vi "Get Device Name.vi"(8 "error in (no error)":errorcluster, 11 "DeviceIndex":u32) -> (0 "error out":errorcluster, 3 "Device Name":string)   [LabVIEW 2014]
doc: "Gets the name of the device specified by <index>"
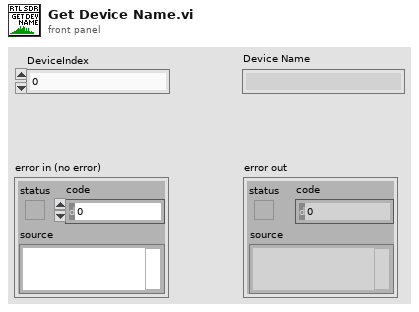
[diagram p1: front panel]
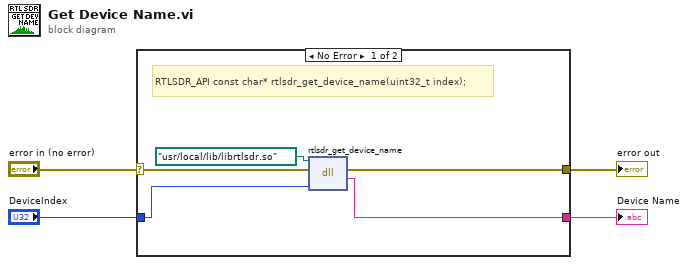
[diagram p0: block diagram]
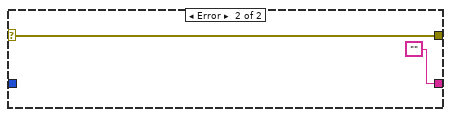
[diagram p2: hidden frame]
diagram:
  n1 = case shown="No Error" "error in (no error)" {
    selector: "error in (no error)" -> [w7 w10]
    tunnel: [w9 ""] -> w4
    tunnel: "DeviceIndex" -> [w8 _]
    tunnel: [w5 w10] -> w1
    frame No Error {
      # "RTLSDR_API const char* rtlsdr_get_device_name(uint32_t index);"
      n2 = dll-call lib="C:/Program Files (x86)/National Instruments/LabVIEW 2016/user.lib/rtlsdr/rtlsdr.*" fn="rtlsdr_get_device_name"(path in=path "/usr/local/lib/librtlsdr.so", error in=w7, "index"=w8) -> (error out=w5:errorcluster, "return type"=w9:string)  [unwired: 2 in, 1 out]
    }
    frame Error {
    }
  }
  "Device Name" <- w4
  "error out" <- w1
